vi "Boiler Controller.vi"(8 "error in":errorcluster, 10 "Notifiers":T1, 11 "Message Queues":T2) -> (0 "error out":errorcluster)   [LabVIEW 2022 SP3]
uses:
  support/Message Queue/All Message Queues.ctl
  support/Message Queue/Message Cluster.ctl
  support/Notifiers/Notifiers.ctl
  support/Message Queue/Message Queue.lvlib
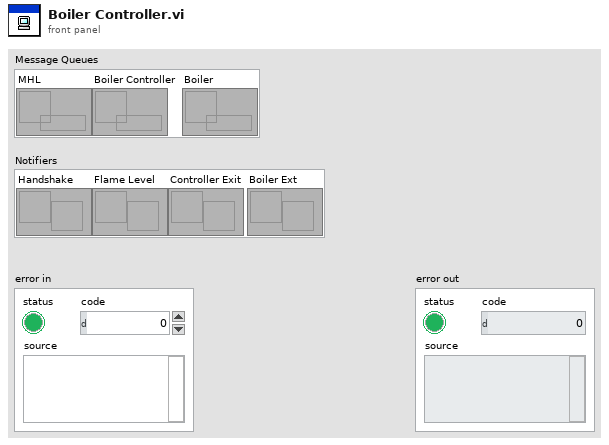
[diagram p1: front panel]
types:
  T1 = typedef "Notifiers.ctl" = cluster{"Handshake":refnum<notifier>, "Flame Level":refnum<notifier>, "Controller Exit":refnum<notifier>, "Boiler Ext":refnum<notifier>}
  T2 = typedef "Message Queue.lvlib/All Message Queues.ctl" = cluster{"MHL":refnum<queue>, "Boiler Controller":refnum<queue>, "Boiler":refnum<queue>}
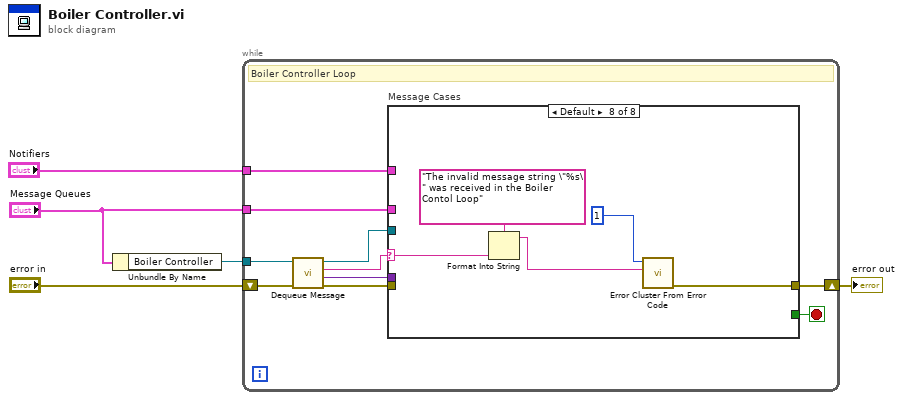
[diagram p0: block diagram]
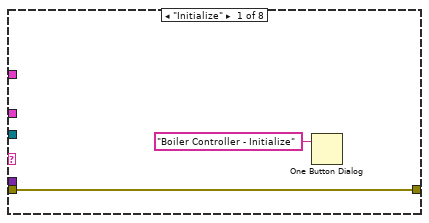
[diagram p2: hidden frame]
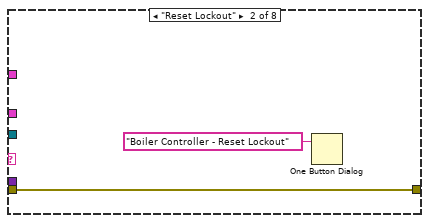
[diagram p3: hidden frame]
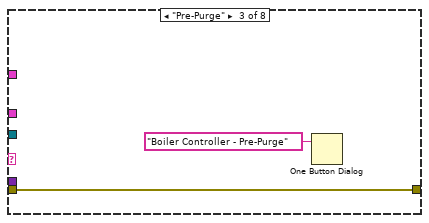
[diagram p4: hidden frame]
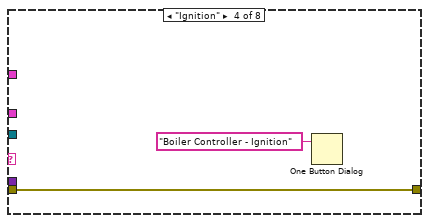
[diagram p5: hidden frame]
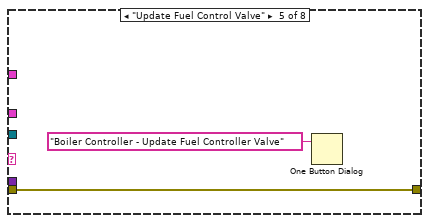
[diagram p6: hidden frame]
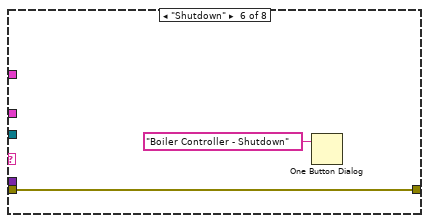
[diagram p7: hidden frame]
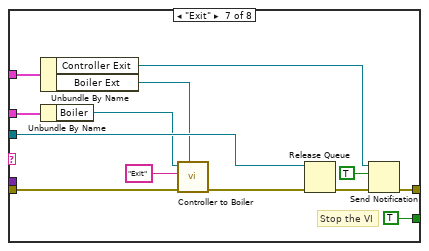
[diagram p8: hidden frame]
diagram:
  n1 = Unbundle By Name("Message Queues") -> ("Boiler Controller"=w5:refnum<queue>)
  n2 = while {
    tunnel: w5 -> [w15]
    shift-right: [w9] -> w3
    shift-left: "error in" -> [w10]
    tunnel: "Notifiers" -> [w7]
    tunnel: "Message Queues" -> [w6]
    stop <- w8 stop-if-true
    # "Boiler Controller Loop"
    n3 = call "Dequeue Message.vi"("error in"=w10, "Message Queue"=w15) -> ("error out"=w11:errorcluster, "Message Data"=w12:variant, "Message"=w14:string, "dup Message Queue"=w13:refnum<queue>)  [unwired: 6 in]
    n4 = case "Message Cases" shown="Default" w14 {
      selector: w14 -> [_ _ _ _ _ _ _ w45]
      tunnel: w13 -> [_ _ _ _ _ _ w40 _]
      tunnel: w12 -> [_ _ _ _ _ _ _ _]
      tunnel: w11 -> [w16 w18 w20 w22 w24 w26 w37 _]
      tunnel: [w16 w18 w20 w22 w24 w26 w30 w43] -> w9
      tunnel: [_ _ _ _ _ _ TRUE _] -> w8
      tunnel: w7 -> [_ _ _ _ _ _ w38 _]
      tunnel: w6 -> [_ _ _ _ _ _ w35 _]
      frame "Initialize" {
        n5 = One Button Dialog(message="Boiler Controller - Initialize") -> ()  [unwired: 1 in, 1 out]
      }
      frame "Reset Lockout" {
        n6 = One Button Dialog(message="Boiler Controller - Reset Lockout") -> ()  [unwired: 1 in, 1 out]
      }
      frame "Pre-Purge" {
        n7 = One Button Dialog(message="Boiler Controller - Pre-Purge") -> ()  [unwired: 1 in, 1 out]
      }
      frame "Ignition" {
        n8 = One Button Dialog(message="Boiler Controller - Ignition") -> ()  [unwired: 1 in, 1 out]
      }
      frame "Update Fuel Control Valve" {
        n9 = One Button Dialog(message="Boiler Controller - Update Fuel Controller Valve") -> ()  [unwired: 1 in, 1 out]
      }
      frame "Shutdown" {
        n10 = One Button Dialog(message="Boiler Controller - Shutdown") -> ()  [unwired: 1 in, 1 out]
      }
      frame "Exit" {
        # "Stop the VI"
        n11 = Unbundle By Name(w38) -> ("Controller Exit"=w29:refnum<notifier>, "Boiler Ext"=w32:refnum<notifier>)
        n12 = Unbundle By Name(w35) -> ("Boiler"=w34:refnum<queue>)
        n13 = call "Controller to Boiler.vi"("Notifier"=w32, "error in"=w37, "Message"="Exit", "Boiler Queue in"=w34) -> ("error out"=w36:errorcluster)  [unwired: 5 in, 2 out]
        n14 = Release Queue(queue=w40, error in (no error)=w36) -> (error out=w31:errorcluster)  [unwired: 1 in, 2 out]
        n15 = Send Notification(notification=TRUE, notifier=w29, error in (no error)=w31) -> (error out=w30:errorcluster)  [unwired: 1 out]
      }
      frame Default {
        n16 = Format Into String(format string="The invalid message string \"%s\" was received in the Boiler Contol Loop", w45) -> (resulting string=w42:string)  [unwired: 2 in, 1 out]
        n17 = call <vilib>:"Error Cluster From Error Code.vi"("error message (\"\")"=w42, "error code (0)"=1) -> ("error out"=w43:errorcluster)  [unwired: 7 in]
      }
    }
  }
  "error out" <- w3
